vi "Actor Core.vi"(8 "error in":errorcluster, 11 "Controller in":refnum<class "Controller.lvclass">) -> (0 "error out":errorcluster, 3 "Actor out":refnum<class "Actor.lvclass">)   [LabVIEW 2013, in "SET Project Editor.lvlib" / "Controller.lvclass"]
doc: "(<B>Filename</B>: Actor Framework.lvlib:Actor.lvclass:Actor Core.vi)\n\nReceives messages to the actor, reacts to them, and initiates any error handling that may shut the actor down.\n\nDescendant classes may override this VI to append parallel tasks for the actor to complete while it handles messages. Overrides use the Call Parent Method node."
uses:
  Controller.lvclass
  <vilib>/ActorFramework/Actor/Actor.lvclass
  Types/Init Cases Enum.ctl
  <vilib>/ActorFramework/Actor/Actor.lvclass/Actor.ctl
  <vilib>/ActorFramework/Message Enqueuer/Message Enqueuer.lvclass/Message Enqueuer.ctl
  Types/Ctrl Refs.ctl
  Controller.lvclass/Controller.ctl
  SET Project Data/Resource Data Class/Resource Data.lvclass
  SET Project Data/Project Data Class/Project Data.lvclass
  views/Project View/Project View.lvclass
  ui view messages/Load View to SubPanel Msg/Load View to SubPanel Msg.lvclass/Load View to SubPanel Msg.ctl
  controller messages/New Project Msg/New Project Msg.lvclass/New Project Msg.ctl
  controller messages/Open Msg/Open Msg.lvclass/Open Msg.ctl
  UI Actor/UI Actor.lvclass
  <vilib>/ActorFramework/Message Enqueuer/Message Priority.ctl
  controller messages/Remove Object Msg/Remove Object Msg.lvclass/Remove Object Msg.ctl
  Controller Messages/Change Selection Msg/Change Selection Msg.lvclass/Change Selection Msg.ctl
  <vilib>/ActorFramework/Message Enqueuer/Init from Existing Queue.vi
  <vilib>/ActorFramework/Message Enqueuer/Enqueue.vi
  <vilib>/ActorFramework/Message Priority Queue/Priority Enqueue.vi
  <vilib>/ActorFramework/Message Enqueuer/Message Enqueuer.lvclass
  controller messages/Shutdown Msg/Shutdown Msg.lvclass
  ui view messages/Load View to SubPanel Msg/Load View to SubPanel Msg.lvclass
  controller messages/New Project Msg/New Project Msg.lvclass
  controller messages/Open Msg/Open Msg.lvclass
  controller messages/UI Update Msg/UI Update Msg.lvclass
  controller messages/Save Msg/Save Msg.lvclass
  controller messages/Export CSV Msg/Export CSV Msg.lvclass
  controller messages/Import CSV Msg/Import CSV Msg.lvclass
  controller messages/Add Language Msg/Add Language Msg.lvclass
  controller messages/Remove Language Msg/Remove Language Msg.lvclass
  controller messages/Apply Language Msg/Apply Language Msg.lvclass
  controller messages/Launch Update Project Wizard Msg/Launch Update Project Wizard Msg.lvclass
  controller messages/Remove Object Msg/Remove Object Msg.lvclass
  Controller Messages/Change Selection Msg/Change Selection Msg.lvclass
  Lib/printf/Core/LV_Printf Core.lvclass
  SET Project Editor.lvlib
panel:
  in  "VI List":string(tree)
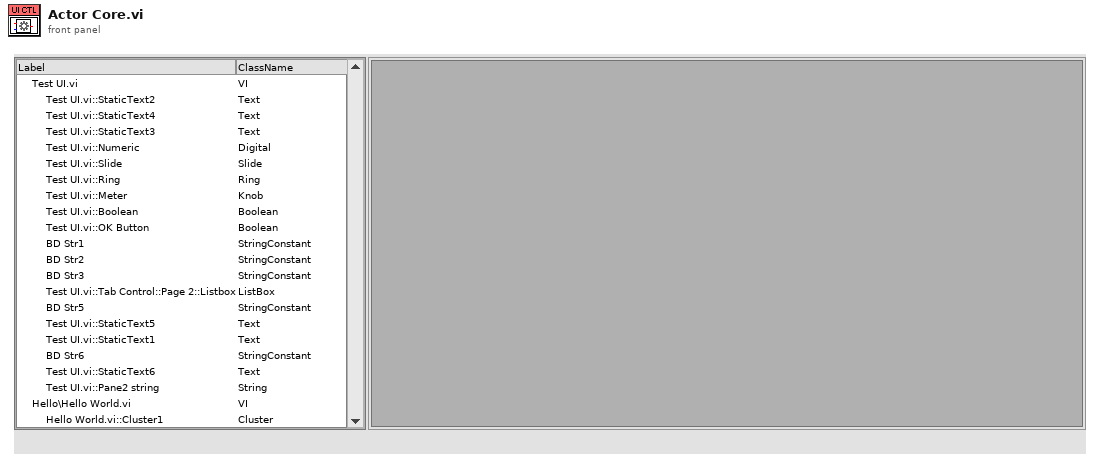
[diagram p1: front panel]
types:
  T1 = typedef "SET Project Editor.lvlib/Controller.lvclass/Init Cases Enum.ctl" = enum16{"Check Unicode", "Init Events and Refs", "Build LangData", "Launch Views", "Init UI", "Error", "Finish"}
  T2 = typedef "SET Project Editor.lvlib/Controller.lvclass/Ctrl Refs.ctl" = cluster{"VI List":refnum<vi>, "SubPnl":refnum<vi>, "Front Panel":refnum<vi>}
  T3 = typedef "Actor Framework.lvlib/Message Enqueuer.lvclass/Message Priority.ctl" = enum16{"Low", "Normal", "High"}
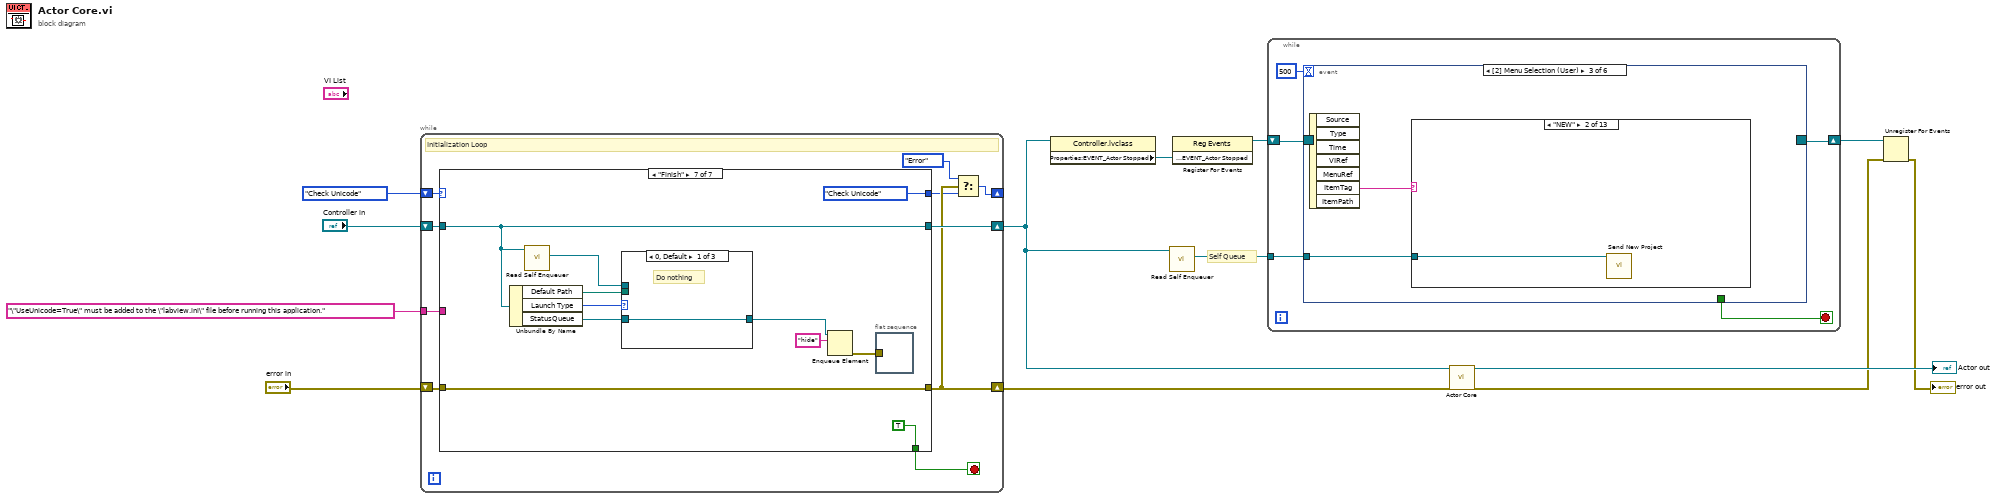
[diagram p0: block diagram]
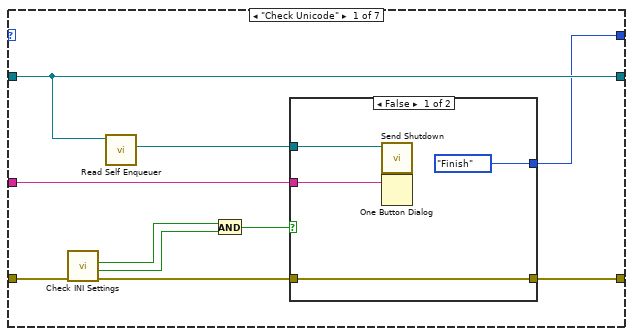
[diagram p2: hidden frame]
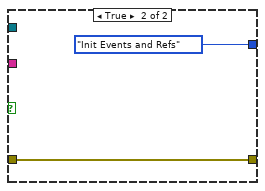
[diagram p3: hidden frame]
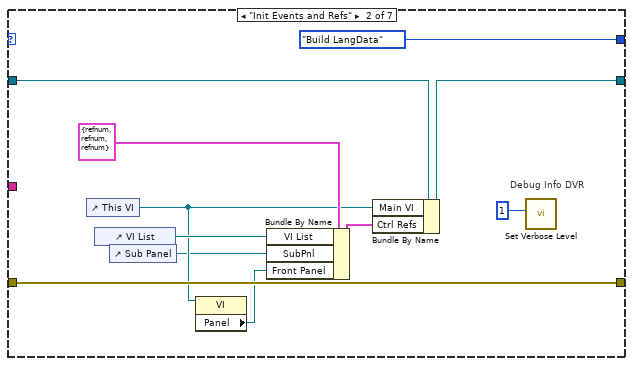
[diagram p4: hidden frame]
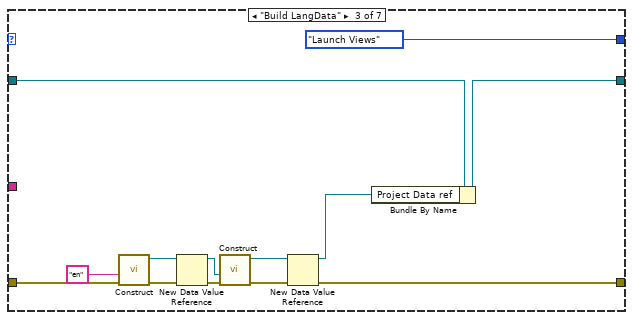
[diagram p5: hidden frame]
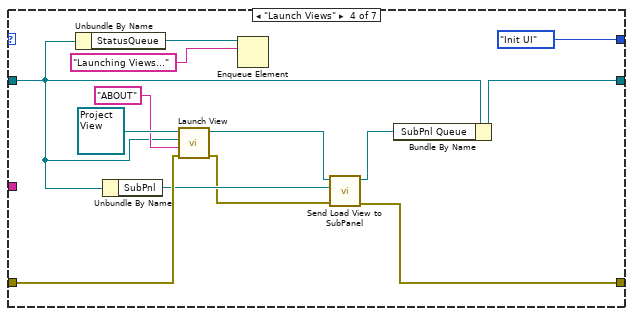
[diagram p6: hidden frame]
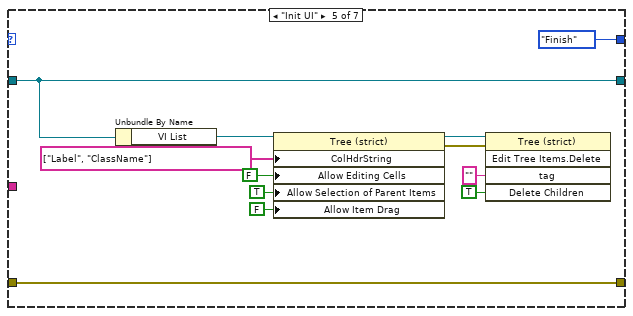
[diagram p7: hidden frame]
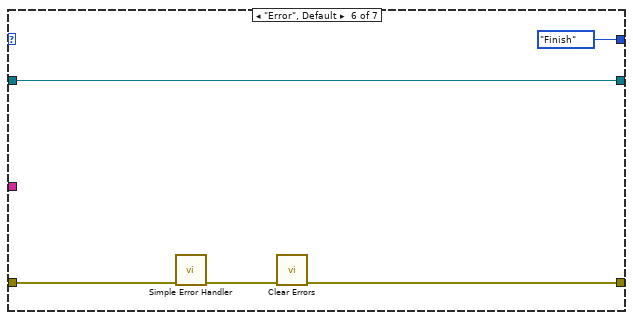
[diagram p8: hidden frame]
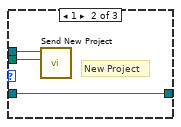
[diagram p9: hidden frame]
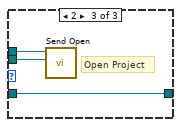
[diagram p10: hidden frame]
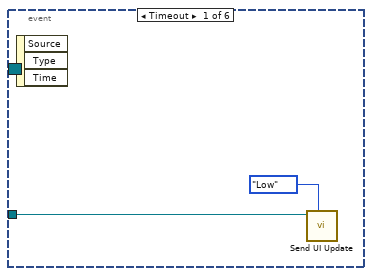
[diagram p11: hidden frame]
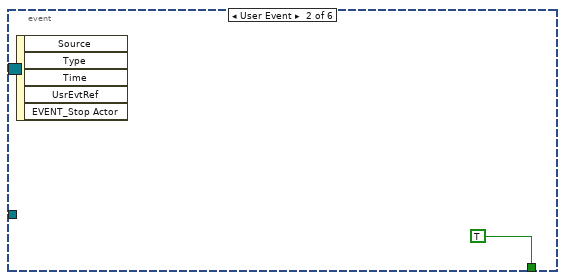
[diagram p12: hidden frame]
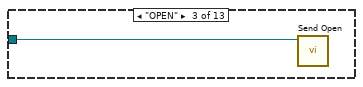
[diagram p14: hidden frame]
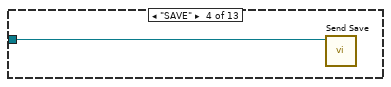
[diagram p15: hidden frame]
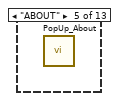
[diagram p16: hidden frame]
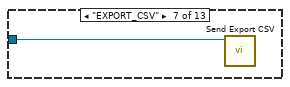
[diagram p18: hidden frame]
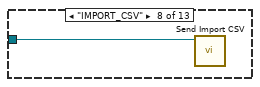
[diagram p19: hidden frame]
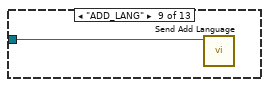
[diagram p20: hidden frame]
diagram:
  # "Self Queue"
  n1 = while {
    shift-right: [w20] -> w6
    shift-left: "Controller in" -> [w22]
    shift-right: [w18] -> w4
    shift-left: "error in" -> [w21]
    shift-right: [w15] -> _
    shift-left: Init_Cases_Enum."Check Unicode" -> [w23]
    tunnel: "\"UseUnicode=True\" must be added to the \"labview.ini\" file before running this application." -> [w14]
    stop <- w19 stop-if-true
    # "Initialization Loop"
    n2 = case shown="\"Finish\"" w23 {
      tunnel: w22 -> [w27 w40 w51 w64 w79 w92 w101]
      tunnel: w21 -> [w33 w46 w52 w76 w78 w91 w97]
      tunnel: [w28 w46 w59 w69 w78 w89 w97] -> w18
      tunnel: [w27 w47 w63 w75 w79 w92 w101] -> w20
      tunnel: [w24 Init_Cases_Enum."Build LangData" Init_Cases_Enum."Launch Views" Init_Cases_Enum."Init UI" Init_Cases_Enum."Finish" Init_Cases_Enum."Finish" Init_Cases_Enum."Check Unicode"] -> w17
      tunnel: [_ _ _ _ _ _ TRUE] -> w19
      tunnel: w14 -> [w25 _ _ _ _ _ _]
      frame "Check Unicode" {
        n3 = call "Check INI Settings.vi"("error in (no error)"=w33) -> ("error out"=w29:errorcluster, "found?"=w32:bool, "value"=w31:bool)  [unwired: 8 in]
        n4 = call <vilib>:"Read Self Enqueuer.vi"("Actor"=w27) -> ("Self Enqueuer"=w26:refnum<class "Message Enqueuer.lvclass">)  [unwired: 10 in]
        n5 = And(x=w31, y=w32) -> (x .and. y?=w30:bool)
        n6 = case shown="False" w30 {
          tunnel: w29 -> [w37 w38]
          tunnel: [w37 w38] -> w28
          tunnel: w26 -> [w36 _]
          tunnel: w25 -> [w35 _]
          tunnel: [Init_Cases_Enum."Finish" ("t") Init_Cases_Enum."Init Events and Refs"] -> w24
          frame False {
            n7 = call "Send Shutdown.vi"("Message Enqueuer"=w36) -> ()  [unwired: 9 in, 2 out]
            n8 = One Button Dialog(message=w35) -> ()  [unwired: 1 in, 1 out]
          }
          frame True {
          }
        }
      }
      frame "Init Events and Refs" {
        # "Debug Info DVR"
        n9 = control-ref of="This VI"() -> (w44:refnum<vi>)
        n10 = control-ref of="VI List"() -> (w49:refnum<vi>)
        n11 = control-ref of="Sub Panel"() -> (w42:refnum<vi>)
        n12 = property class="VI"(reference=w44) -> ("Panel"=w43:refnum<vi>)  [unwired: 1 in, 2 out]
        n13 = Bundle By Name(cluster=T2 {"VI List"=refnum, "SubPnl"=refnum, "Front Panel"=refnum} ("Ctrl Refs"), "VI List"=w49, "SubPnl"=w42, "Front Panel"=w43) -> (w48:T2)
        n14 = Bundle By Name(cluster=w40, "Main VI"=w44, "Ctrl Refs"=w48) -> (w47:refnum<class "Controller.lvclass">)
        n15 = call "Set Verbose Level.vi"("Verbose Level"=1) -> ()  [unwired: 10 in, 1 out]
      }
      frame "Build LangData" {
        n16 = call "Construct.vi"("error in (no error)"=w52, "Default Language"="en") -> ("error out"=w57:errorcluster, "LangFile out"=w56:refnum<class "Resource Data.lvclass">)  [unwired: 8 in]
        n17 = New Data Value Reference(data value=w56, error in=w57) -> (data value reference=w54:refnum<data-value>, error out=w55:errorcluster)
        n18 = call "Construct.vi"("error in (no error)"=w55, "Resource Data ref"=w54) -> ("error out"=w62:errorcluster, "Project Data out"=w61:refnum<class "Project Data.lvclass">)  [unwired: 8 in]
        n19 = New Data Value Reference(data value=w61, error in=w62) -> (data value reference=w60:refnum<data-value>, error out=w59:errorcluster)
        n20 = Bundle By Name(cluster=w51, "Project Data ref"=w60) -> (w63:refnum<class "Controller.lvclass">)
      }
      frame "Launch Views" {
        n21 = Unbundle By Name(w64) -> ("StatusQueue"=w66:refnum<queue>)
        n22 = Unbundle By Name(w64) -> ("SubPnl"=w73:refnum<vi>)
        n23 = call-dynamic "Launch View.vi"("error in (no error)"=w76, "UUID"="ABOUT" ("UID"), "Controller in"=w64, "UI View in"=refnum<class "Project View.lvclass"> refnum ("SET Language Editor.lvlib:Project View.lvclass")) -> ("error out"=w70:errorcluster, "Caller-To-Actor Enqueuer"=w74:refnum<class "Message Enqueuer.lvclass">)  [unwired: 6 in]
        n24 = Enqueue Element(queue=w66, element="Launching Views...") -> ()  [unwired: 2 in, 3 out]
        n25 = call "Send Load View to SubPanel.vi"("error in (no error)"=w70, "SubPnl Refnum"=w73, "Message Enqueuer"=w74) -> ("error out"=w69:errorcluster, "Message Enqueuer out"=w72:refnum<class "Message Enqueuer.lvclass">)  [unwired: 7 in]
        n26 = Bundle By Name(cluster=w64, "SubPnl Queue"=w72) -> (w75:refnum<class "Controller.lvclass">)
      }
      frame "Init UI" {
        n27 = Unbundle By Name(w79) -> ("VI List"=w80:refnum<vi>)
        n28 = property on="Property Node" class="Tree (strict)"(reference=w80, "ColHdrString"=string[] ["Label", "ClassName"] ("Column Header Strings[]"), "Allow Editing Cells"=FALSE, "Allow Selection of Parent Items"=TRUE, "Allow Item Drag"=FALSE ("Drag/Drop:Allow Dragging")) -> (reference out=w85:refnum<vi>, error out=w86:errorcluster)  [unwired: 1 in]
        n29 = invoke class="Tree (strict)" method="Edit Tree Items.Delete"(reference=w85, error in=w86, "tag"="" ("Tag"), "Delete Children"=TRUE ("Delete Children?")) -> ()  [unwired: 1 in, 5 out]
      }
      frame "Error", Default {
        n30 = call <vilib>:"Simple Error Handler.vi"("error in (no error)"=w91) -> ("error out"=w90:errorcluster)  [unwired: 4 in, 4 out]
        n31 = call <vilib>:"Clear Errors.vi"("error in (no error)"=w90) -> ("error out"=w89:errorcluster)  [unwired: 6 in]
      }
      frame "Finish" {
        n32 = Unbundle By Name(w101) -> ("Default Path"=w100:path, "Launch Type"=w99:i32, "StatusQueue"=w95:refnum<queue>)
        n33 = call <vilib>:"Read Self Enqueuer.vi"("Actor"=w101) -> ("Self Enqueuer"=w102:refnum<class "Message Enqueuer.lvclass">)  [unwired: 10 in]
        n34 = case shown="0, Default" w99 {
          tunnel: w102 -> [_ w108 w111]
          tunnel: w100 -> [_ w107 w110]
          tunnel: w95 -> [w105 w106 w109]
          tunnel: [w105 w106 w109] -> w94
          frame 0, Default {
            # "Do nothing"
          }
          frame 1 {
            # "New Project"
            n35 = call "Send New Project.vi"("Path"=w107, "Message Enqueuer"=w108) -> ()  [unwired: 8 in, 2 out]
          }
          frame 2 {
            # "Open Project"
            n36 = call "Send Open.vi"("Path"=w110, "Message Enqueuer"=w111) -> ()  [unwired: 8 in, 2 out]
          }
        }
        n37 = Enqueue Element(queue=w94, element="hide") -> (error out=w96:errorcluster)  [unwired: 2 in, 2 out]
        n38 = flat-sequence {
          tunnel: w96 -> [_]
          frame #0 {
          }
        }
      }
    }
    n39 = Select(t=Init_Cases_Enum."Error", s=w18, f=w17) -> (s? t:f=w15:T1)
  }
  n40 = property class="Controller.lvclass"(reference=w6) -> ("Properties:EVENT_Actor Stopped"=w11:refnum<user-event>)  [unwired: 1 in, 2 out]
  n41 = call <vilib>:"Read Self Enqueuer.vi"("Actor"=w6) -> ("Self Enqueuer"=w5:refnum<class "Message Enqueuer.lvclass">)  [unwired: 10 in]
  n42 = register-events(w11) -> (reference out=w10:refnum<event-registration>)  [unwired: 2 in, 1 out]
  n43 = while {
    shift-right: [w115] -> w9
    shift-left: w10 -> [w116]
    tunnel: w5 -> [w113]
    stop <- w114 stop-if-true
    n44 = event shown="[2] Menu Selection (User)" {
      selector: w116 -> [_ _ _ _ _ _]
      dyn-events: [_ _ _ _ _ _] -> w115
      timeout: 500 -> [_ _ _ _ _ _]
      tunnel: [_ TRUE _ _ _ _] -> w114
      tunnel: w113 -> [w118 _ w120 w132 w139 w140]
      event Timeout {
        n45 = event-data() -> ()  [unwired: 1 in, 3 out]
        n46 = call "Send UI Update.vi"("Message Priority (Normal)"=Message_Priority."Low", "Message Enqueuer"=w118) -> ()  [unwired: 8 in, 2 out]
      }
      event User Event {
        n47 = event-data() -> ()  [unwired: 1 in, 5 out]
      }
      event Menu Selection (User) {
        n48 = event-data() -> ("ItemTag"=w121:string)  [unwired: 1 in, 6 out]
        n49 = case shown="\"NEW\"" w121 {
          tunnel: w120 -> [_ w122 w123 w124 _ _ w125 w126 w127 w128 w129 w130 w131]
          frame Default {
          }
          frame "NEW" {
            n50 = call "Send New Project.vi"("Message Enqueuer"=w122) -> ()  [unwired: 9 in, 2 out]
          }
          frame "OPEN" {
            n51 = call "Send Open.vi"("Message Enqueuer"=w123) -> ()  [unwired: 9 in, 2 out]
          }
          frame "SAVE" {
            n52 = call "Send Save.vi"("Message Enqueuer"=w124) -> ()  [unwired: 9 in, 2 out]
          }
          frame "ABOUT" {
            n53 = call "PopUp_About.vi"() -> ()  [unwired: 11 in, 1 out]
          }
          frame "SAVE_AS" {
          }
          frame "EXPORT_CSV" {
            n54 = call "Send Export CSV.vi"("Message Enqueuer"=w125) -> ()  [unwired: 9 in, 2 out]
          }
          frame "IMPORT_CSV" {
            n55 = call "Send Import CSV.vi"("Message Enqueuer"=w126) -> ()  [unwired: 9 in, 2 out]
          }
          frame "ADD_LANG" {
            n56 = call "Send Add Language.vi"("Message Enqueuer"=w127) -> ()  [unwired: 9 in, 2 out]
          }
          frame "DEL_LANG" {
            n57 = call "Send Remove Language.vi"("Message Enqueuer"=w128) -> ()  [unwired: 9 in, 2 out]
          }
          frame "APPLY_LANG" {
            n58 = call "Send Apply Language.vi"("Message Enqueuer"=w129) -> ()  [unwired: 9 in, 2 out]
          }
          frame "UPDATE_DATA" {
            n59 = call "Send Launch Update Project Wizard.vi"("Message Enqueuer"=w130) -> ()  [unwired: 9 in, 2 out]
          }
          frame "EXIT" {
            n60 = call "Send Shutdown.vi"("Message Enqueuer"=w131) -> ()  [unwired: 9 in, 2 out]
          }
        }
      }
      event "VI List": Shortcut Menu Selection (User) {
        n61 = event-data() -> ("CtlRef"=w133:refnum<vi>, "ItemTag"=w134:string)  [unwired: 1 in, 6 out]
        n62 = case shown="\"DELETE\"" w134 {
          tunnel: w133 -> [_ w137]
          tunnel: w132 -> [_ w136]
          frame "False", Default {
          }
          frame "DELETE" {
            n63 = property class="Tree (strict)"(reference=w137) -> ("Value"=w135:string)  [unwired: 1 in, 2 out]
            n64 = call "Send Remove Object.vi"("UUID"=w135, "Message Enqueuer"=w136) -> ()  [unwired: 8 in, 2 out]
          }
        }
      }
      event "VI List": Value Change {
        n65 = event-data() -> ("NewVal"=w138:string)  [unwired: 1 in, 5 out]
        n66 = call "Send Change Selection.vi"("UID"=w138, "Message Enqueuer"=w139) -> ()  [unwired: 8 in, 2 out]
      }
      event Panel Close? {
        n67 = event-data() -> ()  [unwired: 1 in, 4 out]
        n68 = call "Send Shutdown.vi"("Message Enqueuer"=w140) -> ()  [unwired: 9 in, 2 out]
        n69 = event-data("Discard?"=TRUE) -> ()  [unwired: 1 in, 1 out]
      }
    }
  }
  n70 = call-parent "Actor Core.vi"("error in"=w4, "Actor in"=w6) -> ("error out"=w8:errorcluster, "Actor out"=→"Actor out":refnum<class "Actor.lvclass">)  [unwired: 8 in]
  n71 = Unregister For Events(event registration refnum=w9, error in=w8) -> (error out=→"error out":errorcluster)
